vi "2D_LDA_Time_scale_estimate.vi"(2 "Average Frequency Hz":dbl, 3 "Time":dbl[](array[numeric]), 4 "Velocity 2":dbl[](array[numeric]), 5 "Velocity":dbl[](array[numeric])) -> (0 "Estimated Time Scale BSA2":dbl, 1 "Estimated Time Scale BSA1":dbl)   [LabVIEW 2010]
uses:
  Globals/Meas_global.vi
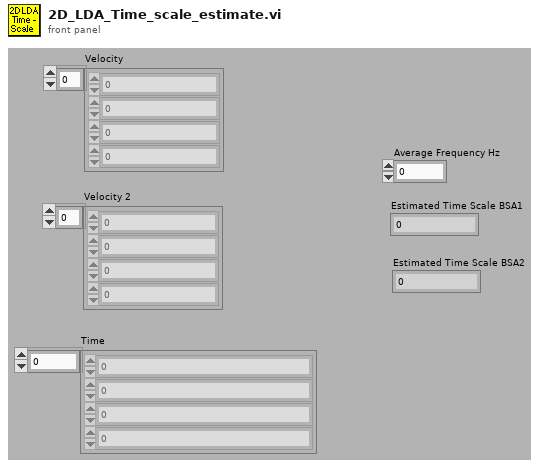
[diagram p1: front panel]
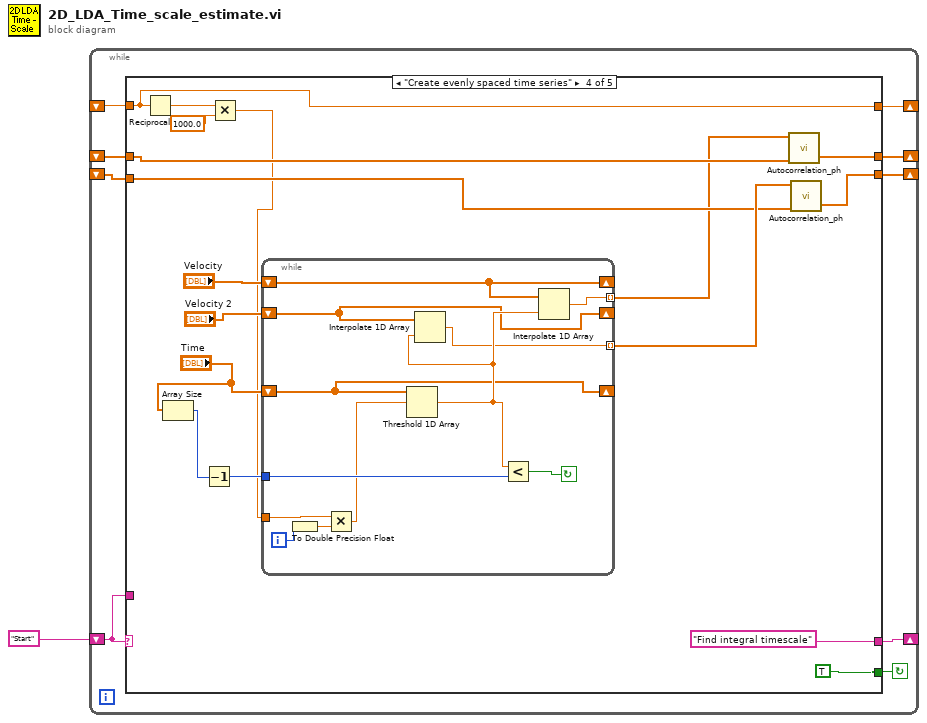
[diagram p0: block diagram]
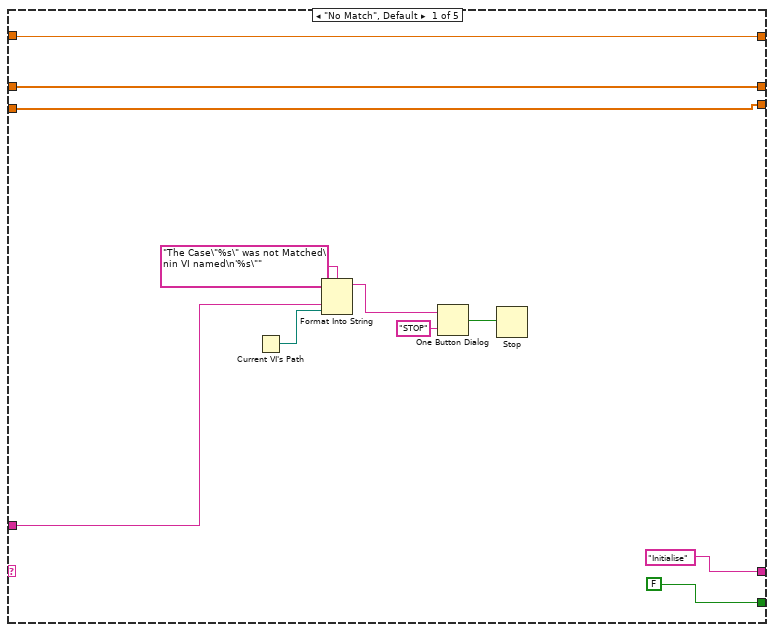
[diagram p2: hidden frame]
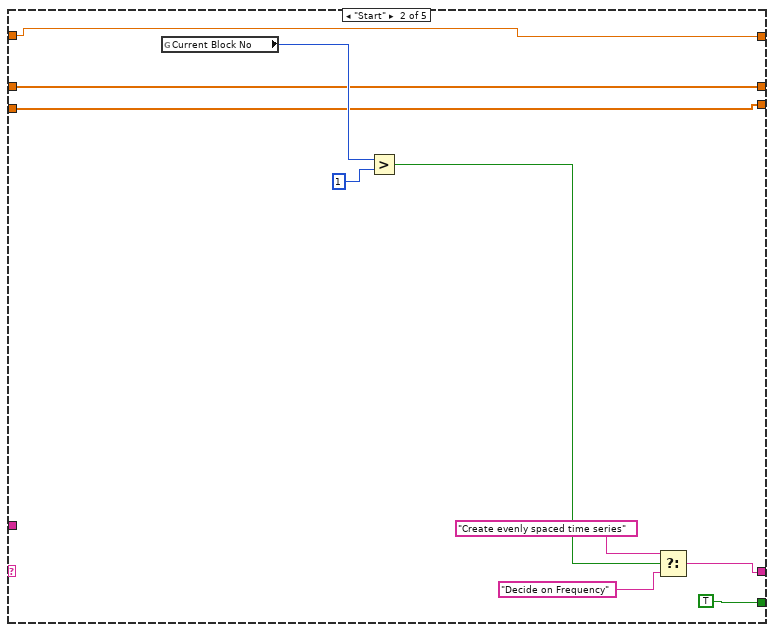
[diagram p3: hidden frame]
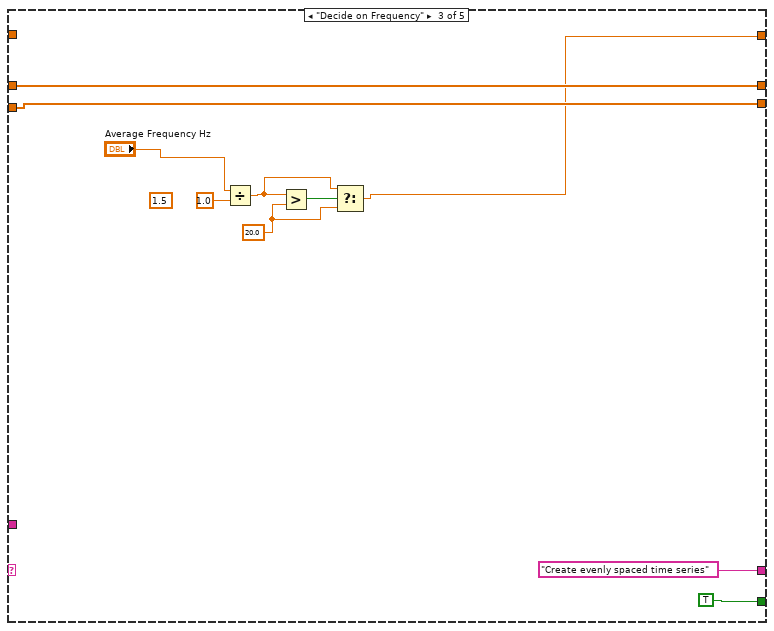
[diagram p4: hidden frame]
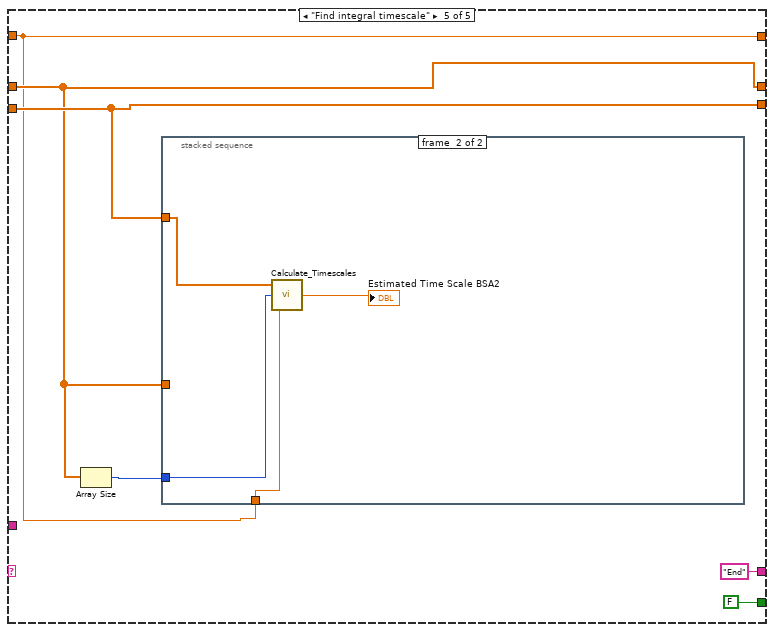
[diagram p5: hidden frame]
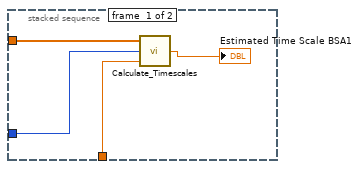
[diagram p6: hidden frame]
diagram:
  n1 = while {
    shift-left: "Start" -> [w8]
    shift-right: [w9] -> _
    shift-right: [w7] -> _
    shift-left: _ -> [w6]
    shift-right: [w5] -> _
    shift-left: _ -> [w4]
    shift-right: [w2] -> _
    shift-left: _ -> [w3]
    stop <- w10 continue-if-true
    n2 = case shown="\"Create evenly spaced time series\"" w8 {
      tunnel: [FALSE TRUE TRUE TRUE FALSE] -> w10
      tunnel: ["Initialise" w30 "Create evenly spaced time series" "Find integral timescale" "End"] -> w9
      tunnel: w8 -> [w16 _ _ _ _]
      tunnel: [w13 w26 w32 w50 w71] -> w7
      tunnel: w6 -> [w13 w26 _ w50 w71]
      tunnel: [w12 w25 w34 w42 w73] -> w5
      tunnel: w4 -> [w12 w25 w34 w49 w73]
      tunnel: w3 -> [w11 w23 w33 w46 w74]
      tunnel: [w11 w23 w33 w45 w74] -> w2
      frame "No Match", Default {
        n3 = Current VI's Path() -> (path=w15:path)
        n4 = Format Into String(format string="The Case\"%s\" was not Matched\nin VI named\n'%s\"" ("Format String"), w16, w15) -> (resulting string=w19:string)  [unwired: 2 in, 1 out]
        n5 = One Button Dialog(message=w19, button name ("OK")="STOP") -> (true=w17:bool)
        n6 = Stop(stop? (T)=w17) -> ()
      }
      frame "Start" {
        n7 = global read "Meas_global.vi" "Current Block No"() -> (w27:i32)
        n8 = Greater?(x=w27, y=1) -> (0:w29:bool)
        n9 = Select(t="Create evenly spaced time series", s=w29, f="Decide on Frequency") -> (s? t:f=w30:string)
      }
      frame "Decide on Frequency" {
        (unwired) 1.5 ("y")
        w36 = 20.0 ("y")
        n10 = Divide(x="Average Frequency Hz", y=1.0) -> (x/y=w37:dbl)
        n11 = Greater?(x=w37, y=w36) -> (0:w38:bool)
        n12 = Select(t=w37, s=w38, f=w36) -> (s? t:f=w32:dbl)
      }
      frame "Create evenly spaced time series" {
        n13 = Reciprocal(x=w50) -> (1/x=w52:dbl)
        n14 = Array Size(array="Time") -> (size(s)=w53:i32)
        n15 = Decrement(x=w53) -> (x-1=w54:i32)
        n16 = Multiply(x=w52, y=1000.0) -> (x*y=w43:dbl)
        n17 = while {
          tunnel: w43 -> [w70]
          tunnel: w54 -> [w69]
          tunnel: [w67] -> w44 mode=indexing
          tunnel: [w64] -> w47 mode=indexing
          shift-right: [w59] -> _
          shift-left: "Velocity" -> [w59]
          shift-right: [w60] -> _
          shift-left: "Velocity 2" -> [w60]
          shift-right: [w61] -> _
          shift-left: "Time" -> [w61]
          i -> [w63]
          stop <- w68 continue-if-true
          n18 = To Double Precision Float(number=w63) -> (double precision float=w62:dbl)
          n19 = Multiply(x=w70, y=w62) -> (x*y=w66:dbl)
          n20 = Threshold 1D Array(2:w66, 3:w61) -> (0:w65:dbl)  [unwired: 1 out]
          n21 = Interpolate 1D Array(1:w65, 2:w60) -> (0:w64:dbl)
          n22 = Less?(x=w65, y=w69) -> (x < y?=w68:bool)
          n23 = Interpolate 1D Array(1:w65, 2:w59) -> (0:w67:dbl)
        }
        n24 = call "Autocorrelation_ph.vi"("X"=w44, "Autocorrelation of X"=w49) -> ("Autocorrelation of X"=w42:dbl[])  [unwired: 3 in, 1 out]
        n25 = call "Autocorrelation_ph.vi"("X"=w47, "Autocorrelation of X"=w46) -> ("Autocorrelation of X"=w45:dbl[])  [unwired: 3 in, 1 out]
      }
      frame "Find integral timescale" {
        n26 = Array Size(array=w73) -> (size(s)=w72:i32)
        n27 = stacked-sequence {
          tunnel: w72 -> [w79 w83]
          tunnel: w73 -> [w80 _]
          tunnel: w74 -> [_ w84]
          tunnel: w71 -> [w78 w82]
          frame #0 {
            n28 = call "Calculate_Timescales.vi"("Sampling Frequency (Hz)"=w78, "Autocorrelation length"=w79, "Autocorrelation"=w80) -> ("Time Scale estimate (s)"=→"Estimated Time Scale BSA1":dbl)
          }
          frame #1 {
            n29 = call "Calculate_Timescales.vi"("Sampling Frequency (Hz)"=w82, "Autocorrelation length"=w83, "Autocorrelation"=w84) -> ("Time Scale estimate (s)"=→"Estimated Time Scale BSA2":dbl)
          }
        }
      }
    }
  }
